vi "Set DataArray (String).vi"(8 "error in":errorcluster, 10 "Data":string[][](array[string]), 11 "DataGridView in":refnum<class "DataGridView.lvclass">) -> (0 "error out":errorcluster, 3 "DataGridView out":refnum<class "DataGridView.lvclass">)   [LabVIEW 2016, in "DataGrid.lvlib" / "DataGridView.lvclass"]
uses:
  <userlib>/LabVIEWdotNetDataGrid/source/DataGridView/DataGridView.lvclass
  <userlib>/LabVIEWdotNetDataGrid/source/DataGridView/DataGridView.lvclass/DataGridView.ctl
  System.Windows.Forms
  <userlib>/LabVIEWdotNetDataGrid/source/DataTable/Add Rows (String).vi
  <userlib>/LabVIEWdotNetDataGrid/source/DataTable/DataTable.lvclass
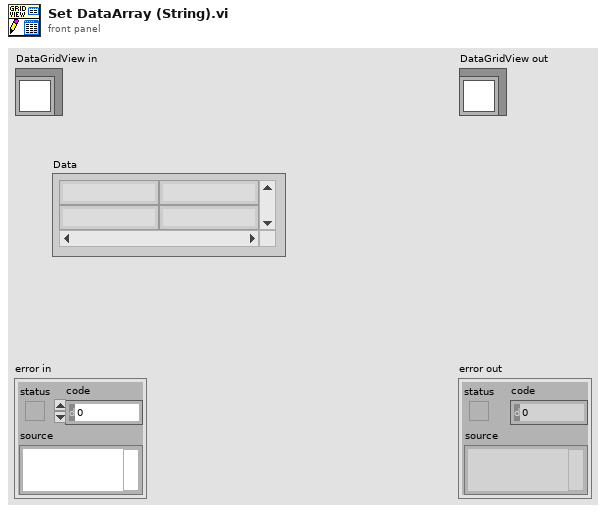
[diagram p1: front panel]
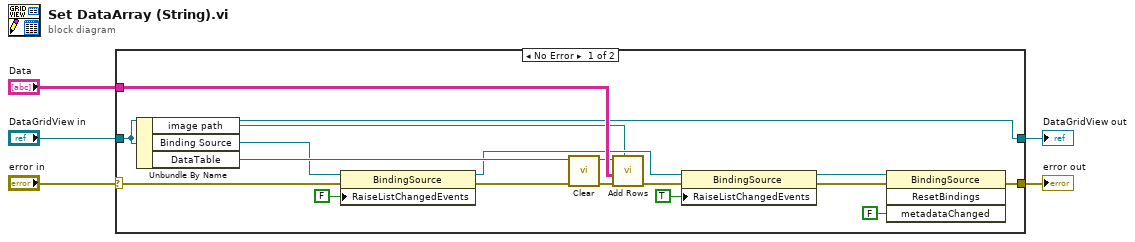
[diagram p0: block diagram]
diagram:
  n1 = case shown="No Error" "error in" {
    selector: "error in" -> [w15 w23]
    tunnel: [w12 w23] -> w4
    tunnel: [w21 w24] -> w2
    tunnel: "DataGridView in" -> [w21 w24]
    tunnel: "Data" -> [w22 _]
    frame No Error {
      n2 = Unbundle By Name(w21) -> ("image path"=w6:path, "Binding Source"=w17:refnum<k24>, "DataTable"=w19:refnum<class "DataTable.lvclass">)
      n3 = property class="BindingSource"(reference=w17, error in=w15, "RaiseListChangedEvents"=FALSE) -> (reference out=w16:refnum<k24>, error out=w14:errorcluster)
      n4 = call <userlib>:"Clear.vi"("error in (no error)"=w14, "DataTable in"=w19) -> ("error out"=w20:errorcluster, "DataTable out"=w18:refnum<class "DataTable.lvclass">)  [unwired: 8 in]
      n5 = call-poly <userlib>:"Add Rows.vi"("image path"=w6, "error in (no error)"=w20, "String Data"=w22, "DataTable in"=w18) -> ("error out"=w13:errorcluster)  [unwired: 6 in, 1 out]
      n6 = property class="BindingSource"(reference=w16, error in=w13, "RaiseListChangedEvents"=TRUE) -> (reference out=w9:refnum<k24>, error out=w10:errorcluster)
      n7 = invoke class="BindingSource" method="ResetBindings"(reference=w9, error in=w10, "metadataChanged"=FALSE) -> (error out=w12:errorcluster)  [unwired: 1 in, 3 out]
    }
    frame Error {
    }
  }
  "error out" <- w4
  "DataGridView out" <- w2
